vi "ep_Scaling Ratio.vi"(8 "error in (no error)":errorcluster, 9 "system info in":refnum<class "EP System Info.lvclass">, 10 "CT/VT ratio":cluster{"primary":dbl, "secondary":dbl}[](array[cluster]), 11 "waveforms in":waveform(dbl)[](array[waveform])) -> (0 "error out":errorcluster, 1 "system info out":refnum<class "EP System Info.lvclass">, 3 "waveforms out":waveform(dbl)[](array[waveform]))   [LabVIEW 2014, in "NI_EP_Power Quality.lvlib"]
uses:
  <vilib>/addons/Electrical Power/PQ/NI_EP_Power Quality.lvlib
  <vilib>/addons/Electrical Power/PQ/Common/Classes/System Info/EP System Info.lvclass
panel:
  # ":"
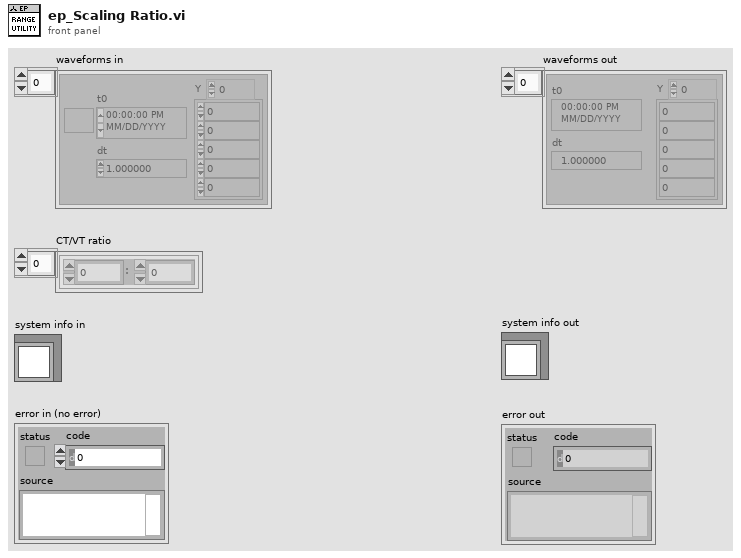
[diagram p1: front panel]
types:
  T1 = typedef "NI_EP_Power Quality.lvlib/ep_Channel Sensitivity.ctl" = cluster{"3-phase system ID":string, "sensitivity":dbl[]}
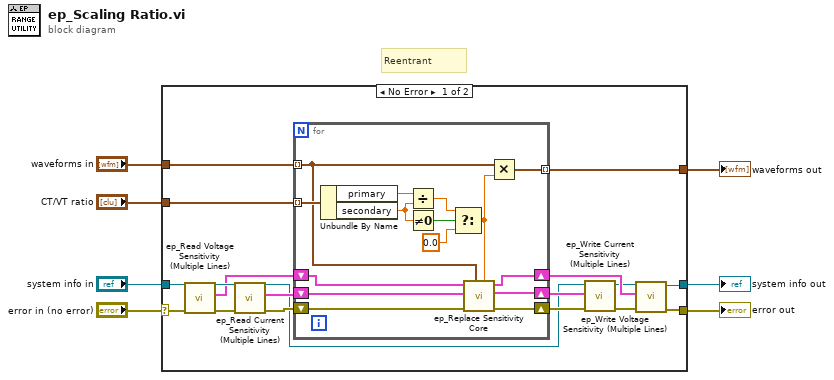
[diagram p0: block diagram]
diagram:
  # "Reentrant"
  n1 = case shown="No Error" "error in (no error)" {
    selector: "error in (no error)" -> [w19 w43]
    tunnel: "waveforms in" -> [w25 w41]
    tunnel: "system info in" -> [w23 w42]
    tunnel: [w8 w42] -> w5
    tunnel: [w13 w43] -> w4
    tunnel: "CT/VT ratio" -> [w18 _]
    tunnel: [w17 w41] -> w1
    frame No Error {
      n2 = call <vilib>:"ep_Read Voltage Sensitivity (Multiple Lines).vi"("error in (no error)"=w19, "system info in"=w23) -> ("error out"=w21:errorcluster, "voltage sensitivity (multiline)"=w16:T1[], "system info out"=w24:refnum<class "EP System Info.lvclass">)  [unwired: 7 in]
      n3 = call <vilib>:"ep_Read Current Sensitivity (Multiple Lines).vi"("error in (no error)"=w21, "system info in"=w24) -> ("error out"=w20:errorcluster, "current sensitivity (multiline)"=w22:T1[], "system info out"=w10:refnum<class "EP System Info.lvclass">)  [unwired: 7 in]
      n4 = for {
        shift-right: [w29] -> w15
        shift-left: w20 -> [w32]
        tunnel: w25 -> [w31] mode=indexing
        tunnel: w18 -> [w35] mode=indexing
        tunnel: [w34] -> w17 mode=indexing
        shift-right: [w27] -> w12
        shift-left: w16 -> [w28]
        shift-right: [w26] -> w11
        shift-left: w22 -> [w33]
        n5 = Unbundle By Name(w35) -> ("primary"=w40:dbl, "secondary"=w39:dbl)
        n6 = Divide(x=w40, y=w39) -> (x/y=w37:dbl)
        n7 = Not Equal To 0?(x=w39) -> (x != 0?=w38:bool)
        n8 = Select(t=w37, s=w38, f=0.0) -> (s? t:f=w30:dbl)
        n9 = call <vilib>:"ep_Replace Sensitivity Core.vi"("sensitivity"=w30, "waveform"=w31, "error in (no error)"=w32, "current sensitivity (multiline) in"=w33, "voltage sensitivity (multiline) in"=w28) -> ("error out"=w29:errorcluster, "current sensitivity (multiline) out"=w26:T1[], "voltage sensitivity (multiline) out"=w27:T1[])  [unwired: 4 in]
        n10 = Multiply(x=w31, y=w30) -> (x*y=w34:waveform(dbl))
      }
      n11 = call <vilib>:"ep_Write Current Sensitivity (Multiple Lines).vi"("error in (no error)"=w15, "current sensitivity (multiline)"=w11, "system info in"=w10) -> ("error out"=w14:errorcluster, "system info out"=w9:refnum<class "EP System Info.lvclass">)  [unwired: 7 in]
      n12 = call <vilib>:"ep_Write Voltage Sensitivity (Multiple Lines).vi"("error in (no error)"=w14, "voltage sensitivity (multiline)"=w12, "system info in"=w9) -> ("error out"=w13:errorcluster, "system info out"=w8:refnum<class "EP System Info.lvclass">)  [unwired: 7 in]
    }
    frame Error {
    }
  }
  "error out" <- w4
  "system info out" <- w5
  "waveforms out" <- w1
